vi "TSP-Link Group.vi"(8 "error in":errorcluster, 9 "Group (0)":u32 max=64, 10 "Node In":string, 11 "VISA resource name":refnum<visa-resource-name>) -> (0 "error out":errorcluster, 2 "Node Out":string, 3 "VISA resource name out":refnum<visa-resource-name>, 4 "Command String":string)   [LabVIEW 2012, in "Keithley 2600 Series.lvlib"]
doc: "This VI sets the TSP-Link group number of the selected node.\n\n<b>Functions and Attributes used</b>\ntsplink.group\n\nNote:\nTSP-Link feature is not supported with Keithley 2604B, 2614B, 2634B."
uses:
  Keithley 2600 Series.lvlib
  Private/GlobalVariables.vi
panel:
  # "(c) 2008 Keithley Instruments, Inc.  ALL RIGHTS RESERVED."
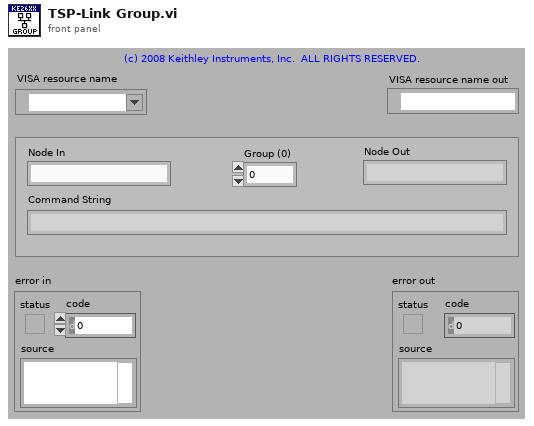
[diagram p1: front panel]
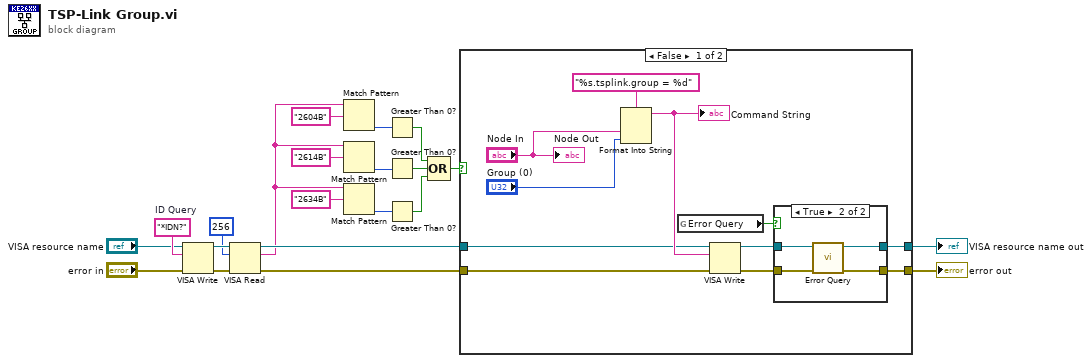
[diagram p0: block diagram]
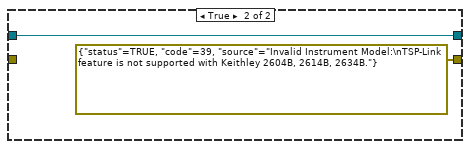
[diagram p3: hidden frame]
diagram:
  w17 = "*IDN?"  # ID Query
  n1 = VISA Write(VISA resource name="VISA resource name", write buffer=w17, error in (no error)="error in") -> (VISA resource name out=w19:refnum<visa-resource-name>, error out=w18:errorcluster)  [unwired: 1 out]
  n2 = VISA Read(VISA resource name=w19, byte count=u32 256, error in (no error)=w18) -> (VISA resource name out=w14:refnum<visa-resource-name>, read buffer=w3:string, error out=w13:errorcluster)  [unwired: 1 out]
  n3 = Match Pattern(string=w3, regular expression="2604B" ("y")) -> (offset past match=w9:i32)  [unwired: 1 in, 3 out]
  n4 = Match Pattern(string=w3, regular expression="2614B" ("y")) -> (offset past match=w8:i32)  [unwired: 1 in, 3 out]
  n5 = Match Pattern(string=w3, regular expression="2634B" ("y")) -> (offset past match=w7:i32)  [unwired: 1 in, 3 out]
  n6 = Greater Than 0?(x=w9) -> (x > 0?=w6:bool)
  n7 = Greater Than 0?(x=w8) -> (x > 0?=w5:bool)
  n8 = Greater Than 0?(x=w7) -> (x > 0?=w4:bool)
  n9 = Compound Arithmetic op=OR(w6, w5, w4) -> (w2:bool)
  n10 = case shown="False" w2 {
    tunnel: [w26 w40] -> w21
    tunnel: [w25 errorcluster {"status"=TRUE, "code"=39, "source"="Invalid Instrument Model:\nTSP-Link feature is not supported with Keithley 2604B, 2614B, 2634B."} ("error out")] -> w20
    tunnel: w14 -> [w23 w40]
    tunnel: w13 -> [w22 _]
    frame False {
      n11 = Format Into String(format string="%s.tsplink.group = %d", "Node In", "Group (0)") -> (resulting string=w24:string)  [unwired: 2 in, 1 out]
      "Command String" <- w24
      n12 = global read "GlobalVariables.vi" "Error Query"() -> (w29:bool)
      n13 = VISA Write(VISA resource name=w23, write buffer=w24, error in (no error)=w22) -> (VISA resource name out=w28:refnum<visa-resource-name>, error out=w27:errorcluster)  [unwired: 1 out]
      n14 = case shown="True" w29 {
        tunnel: w28 -> [w34 w38]
        tunnel: w27 -> [w33 w37]
        tunnel: [w34 w36] -> w26
        tunnel: [w33 w35] -> w25
        frame False {
        }
        frame True {
          n15 = call "Error Query.vi"("error in (no error)"=w37, "VISA resource name"=w38) -> ("error out"=w35:errorcluster, "VISA resource name out"=w36:refnum<visa-resource-name>)  [unwired: 8 out]
        }
      }
      "Node Out" <- "Node In"
    }
    frame True {
    }
  }
  "VISA resource name out" <- w21
  "error out" <- w20
